vi "stepwise retract.vi"(7 "reset motion":T1=enum."fast", 8 "error in":errorcluster, 10 "retract distance (um)":dbl=100.0, 11 "manp in":T2={"Actuator COM"="COM14", "Actuator type"=enum."Scientifica"}) -> (0 "error out":errorcluster, 3 "manip out":T2={"Actuator COM"="COM14", "Actuator type"=enum."Scientifica"})   [LabVIEW 2015]
uses:
  controls/scope_motion.ctl
  pipette cleaning/pressure box/cleaning_soft/controls/scientifica_commands.ctl
  pipette cleaning/pressure box/cleaning_soft/controls/actuator_type.ctl
  pipette cleaning/pressure box/cleaning_soft/controls/actuator_cluster.ctl
panel:
  in  "retract step size (um)":dbl=5.0
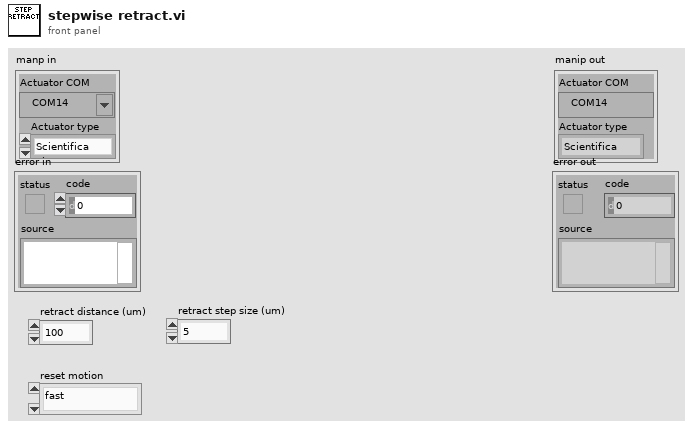
[diagram p1: front panel]
types:
  T1 = typedef "scope_motion.ctl" = enum16{"superSlow", "fast", "slow", "find slice speed", "slow_dualPatch"}
  T2 = typedef "actuator_cluster.ctl" = cluster{"Actuator COM":refnum<visa-resource-name>, "Actuator type":T3}
  T3 = typedef "actuator_type.ctl" = enum16{"Scientifica", "Sutter", "Demo", "Off"}
  T4 = typedef "scientifica_commands.ctl" = enum16{"ANGLE", "INSET", "FIRST", "ZERO", "Pz", "P", "absz", "ACC", "TOP", "STOP", "rel", "relz", "abs", "IN", "vj", "APROACH", "OBJS", "OBJU", "OUT", "OBJ", "OBJL", "SET", "OBJD", "STEP", "SETSTEP", "S", "UUX", "UUY", "UUZ"}
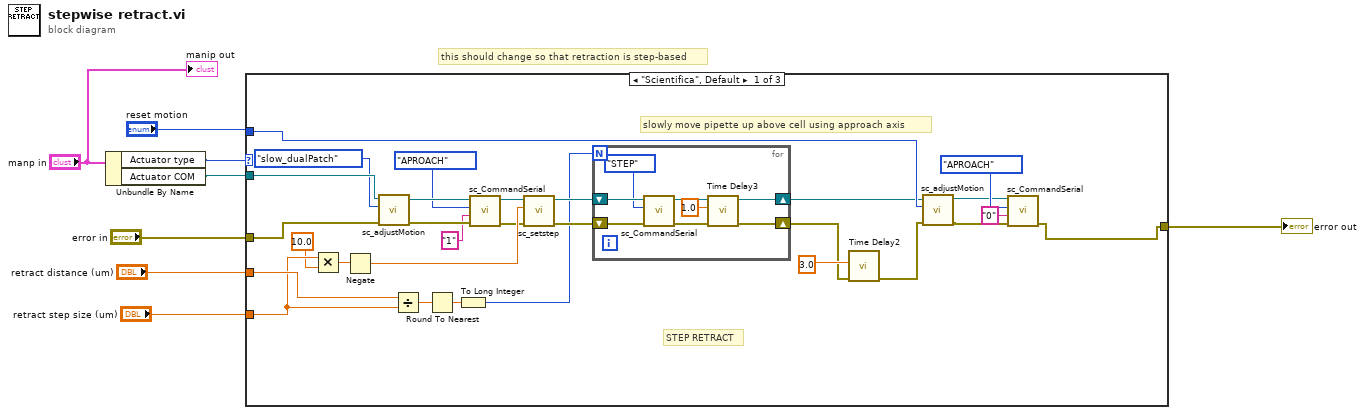
[diagram p0: block diagram]
diagram:
  # "this should change so that retraction is step-based"
  n1 = Unbundle By Name("manp in") -> ("Actuator type"=w7:T3, "Actuator COM"=w6:refnum<visa-resource-name>)
  n2 = case shown="\"Scientifica\", Default" w7 {
    tunnel: w6 -> [w34 _ _]
    tunnel: "retract distance (um)" -> [w37 _ _]
    tunnel: "error in" -> [w36 w45 w46]
    tunnel: [w35 w45 w46] -> w3
    tunnel: "reset motion" -> [w33 _ _]
    tunnel: "retract step size (um)" -> [w32 _ _]
    frame "Scientifica", Default {
      # "STEP RETRACT"
      # "slowly move pipette up above cell using approach axis"
      n3 = Multiply(x=w32, y=10.0) -> (x*y=w16:dbl)
      n4 = Negate(x=w16) -> (-x=w15:dbl)
      n5 = call "sc_adjustMotion.vi"("error in (no error)"=w36, "motion"=scope_motion."slow_dualPatch", "VISA handle"=w34) -> ("error out"=w19:errorcluster, "Dup. VISA handle"=w20:refnum<visa-resource-name>)  [unwired: 7 in]
      n6 = Divide(x=w37, y=w32) -> (x/y=w11:dbl)
      n7 = Round To Nearest(number=w11) -> (nearest integer value=w10:dbl)
      n8 = To Long Integer(number=w10) -> (32bit integer=w9:i32)
      n9 = call "sc_CommandSerial.vi"("error in (no error)"=w19, "argument"="1", "Scientifica commands"=scientifica_commands."APROACH", "VISA handle"=w20) -> ("error out"=w13:errorcluster, "Dup. VISA handle"=w14:refnum<visa-resource-name>)  [unwired: 4 in, 2 out]
      n10 = call "sc_setstep.vi"("error in"=w13, "step distance (steps)"=w15, "VISA in"=w14) -> ("error out"=w24:errorcluster, "VISA out"=w25:refnum<visa-resource-name>)  [unwired: 6 in, 1 out]
      n11 = for {
        N: w9 -> [_]
        shift-right: [w42] -> w23
        shift-left: w25 -> [w44]
        shift-right: [w39] -> w12
        shift-left: w24 -> [w43]
        n12 = call "sc_CommandSerial.vi"("error in (no error)"=w43, "Scientifica commands"=scientifica_commands."STEP", "VISA handle"=w44) -> ("error out"=w40:errorcluster, "Dup. VISA handle"=w42:refnum<visa-resource-name>)  [unwired: 5 in, 2 out]
        n13 = call "Time Delay3"("error in (no error)"=w40, "Delay Time (s)"=1.0) -> ("error out"=w39:errorcluster)  [unwired: 9 in]
      }
      n14 = call "Time Delay2"("error in (no error)"=w12, "Delay Time (s)"=3.0) -> ("error out"=w21:errorcluster)  [unwired: 9 in]
      n15 = call "sc_adjustMotion.vi"("error in (no error)"=w21, "motion"=w33, "VISA handle"=w23) -> ("error out"=w26:errorcluster, "Dup. VISA handle"=w27:refnum<visa-resource-name>)  [unwired: 7 in]
      n16 = call "sc_CommandSerial.vi"("error in (no error)"=w26, "argument"="0", "Scientifica commands"=scientifica_commands."APROACH", "VISA handle"=w27) -> ("error out"=w35:errorcluster)  [unwired: 4 in, 3 out]
    }
    frame "Sutter" {
    }
    frame "Demo" {
    }
  }
  "error out" <- w3
  "manip out" <- "manp in"
